vi "GlobalCalLampInfo.vi"() -> ()   [LabVIEW 2019]
panel:
  in  "Cal-Info":T1(array[cluster])=[{"Element"="Ne", "Wavelength"=808.2458, "CalWidth"=3.0}, {"Element"="Ne", "Wavelength"=794.3181, "CalWidth"=10.0}, {"Element"="Ne", "Wavelength"=743.8898, "CalWidth"=15.0}, {"Element"="Ne", "Wavelength"=724.5167, "CalWidth"=6.0}, {"Element"="Ne", "Wavelength"=717.3938, "CalWidth"=6.0}, {"Element"="Ne", "Wavelength"=703.2413, "CalWidth"=9.0}, {"Element"="Ne", "Wavelength"=692.9467, "CalWidth"=9.0}, {"Element"="Ne", "Wavelength"=671.7043, "CalWidth"=3.0}, {"Element"="Ne", "Wavelength"=667.8276, "CalWidth"=3.0}, {"Element"="Ne", "Wavelength"=659.8953, "CalWidth"=6.0}, {"Element"="Ne", "Wavelength"=653.2882, "CalWidth"=2.1}, {"Element"="Ne", "Wavelength"=650.6528, "CalWidth"=2.2}, {"Element"="Ne", "Wavelength"=640.2246, "CalWidth"=1.5}, {"Element"="Ne", "Wavelength"=638.2991, "CalWidth"=1.4}, {"Element"="Ne", "Wavelength"=633.4428, "CalWidth"=2.8}, {"Element"="Ne", "Wavelength"=632.81646, "CalWidth"=0.5}, {"Element"="Hg", "Wavelength"=579.22, "CalWidth"=1.8}, {"Element"="Hg", "Wavelength"=577.11, "CalWidth"=1.8}, {"Element"="Hg", "Wavelength"=546.22, "CalWidth"=20.0}, {"Element"="Hg", "Wavelength"=435.95, "CalWidth"=10.0}, {"Element"="Hg", "Wavelength"=407.89, "CalWidth"=2.4}, {"Element"="Hg", "Wavelength"=404.77, "CalWidth"=2.4}, {"Element"="Hg", "Wavelength"=366.43, "CalWidth"=0.9}, {"Element"="Hg", "Wavelength"=365.59, "CalWidth"=0.3}, {"Element"="Hg", "Wavelength"=365.12, "CalWidth"=0.3}] {"CalWidth" format="%.4f"; "Wavelength" format="%.4f"}
  # "nm"
  # "+-"
  # "nm"
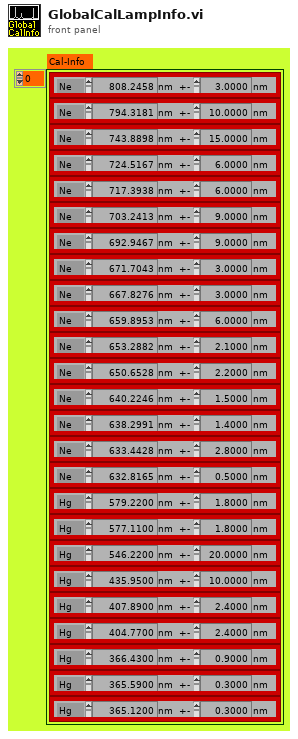
[diagram p1: front panel]
types:
  T1 = cluster{"Element":string, "Wavelength":dbl, "CalWidth":dbl}[]
diagram:
